vi "In Range [0-y].vi"(8 "X":i32, 9 "Y (0)":u32) -> (1 "In Range?":bool)   [LabVIEW 2012]
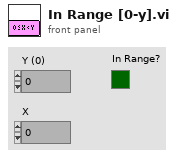
[diagram p1: front panel]
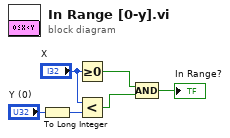
[diagram p0: block diagram]
diagram:
  n1 = To Long Integer(number="Y (0)") -> (32bit integer=w1:i32)
  n2 = Greater Or Equal To 0?(x="X") -> (x >= 0?=w4:bool)
  n3 = Less?(x="X", y=w1) -> (x < y?=w3:bool)
  n4 = Compound Arithmetic op=AND(w4, w3) -> (→"In Range?":bool)
